vi "UpdateGetTerm.vi"(1 "State In":T1 {"BlockNodeState"."Draw Style" items=["FunctionBlock", "ExpressVI", "Variable", "Elemental I/O", "32x32 Icon", "FunctionBlockCompact"]; "BlockNodeState"."Terminal Data"."Terminal Flags" format="%.0b"}) -> (0 "State Out":T1 {"BlockNodeState"."Draw Style" items=["FunctionBlock", "ExpressVI", "Variable", "Elemental I/O", "32x32 Icon", "FunctionBlockCompact"]; "BlockNodeState"."Terminal Data"."Terminal Flags" format="%.0b"})   [LabVIEW 2017, in "Get DDT Properties.lvlib"]
uses:
  <vilib>/express/express signal manip/GetorSetDDTAttributes/Get DDT Attributes/Get DDT Properties.lvlib
  <vilib>/express/express signal manip/GetorSetDDTAttributes/Get DDT Attributes/State.ctl
  <vilib>/BlockNodeSupport/BlockNodeState.ctl
  <vilib>/BlockNodeSupport/TerminalData.ctl
  <vilib>/picture/picture.llb/imagedata.ctl
  <vilib>/express/express signal manip/GetorSetDDTAttributes/Shared VIs/Attributes data.ctl
  <vilib>/express/express signal manip/GetorSetDDTAttributes/Shared VIs/Input.ctl
  <vilib>/express/express signal manip/GetorSetDDTAttributes/Shared VIs/Attributes name.ctl
  <vilib>/express/express signal manip/GetorSetDDTAttributes/Shared VIs/XDimension.ctl
  <vilib>/express/express signal manip/GetorSetDDTAttributes/Shared VIs/TimeType.ctl
  <vilib>/express/express signal manip/GetorSetDDTAttributes/Shared VIs/GetSetShared.lvlib
  <vilib>/express/express signal manip/GetorSetDDTAttributes/Get DDT Attributes/Get DDT Properties.xnode
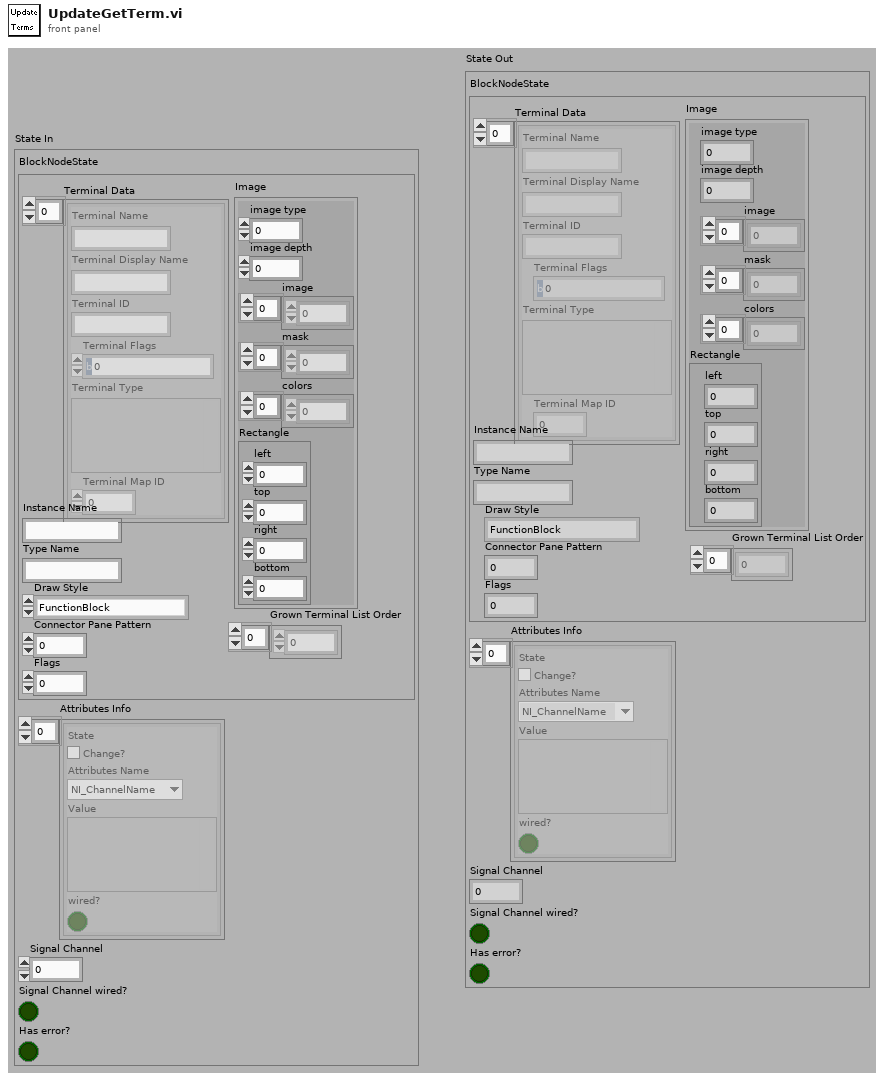
[diagram p1: front panel]
types:
  T1 = typedef "Get DDT Properties.lvlib/Get DDT Properties.xnode/State.ctl" = cluster{"BlockNodeState":T2, "Attributes Info":T5[], "Signal Channel":u32, "Signal Channel wired?":bool, "Has error?":bool}
  T2 = typedef "BlockNodeState.ctl" = cluster{"Terminal Data":T3[], "Instance Name":string, "Type Name":string, "Draw Style":i32, "Connector Pane Pattern":i32, "Flags":i32, "Grown Terminal List Order":i32[], "Image":T4}
  T3 = typedef "TerminalData.ctl" = cluster{"Terminal Name":string, "Terminal Display Name":string, "Terminal ID":string, "Terminal Flags":i32, "Terminal Type":variant, "Terminal Map ID":i32}
  T4 = typedef "imagedata.ctl" = cluster{"image type":i32, "image depth":i32, "image":u8[], "mask":u8[], "colors":u32[], "Rectangle":cluster{"left":i16, "top":i16, "right":i16, "bottom":i16}}
  T5 = typedef "GetSetShared.lvlib/Attributes data.ctl" = cluster{"State":T6, "Attributes Name":T7, "Value":variant, "wired?":bool}
  T6 = typedef "GetSetShared.lvlib/Input.ctl" = bool
  T7 = typedef "GetSetShared.lvlib/Attributes name.ctl" = enum16{"NI_ChannelName", "NI_ExpIsRelativeTime", "NI_ExpTimeStamp", "NI_ExpStartTimeStamp", "NI_ExpXDimension", "NI_UnitDescription"}
  T8 = cluster{"Terminal Name":string, "Terminal Display Name":string, "Terminal ID":string, "Terminal Flags":i32, "Terminal Type":variant, "Terminal Map ID":i32}
  T9 = typedef "GetSetShared.lvlib/XDimension.ctl" = enum16{"No Unit [-]", "Time [sec]", "Frequency [Hz]"}
  T10 = typedef "GetSetShared.lvlib/TimeType.ctl" = enum16{"Absolute", "Relative"}
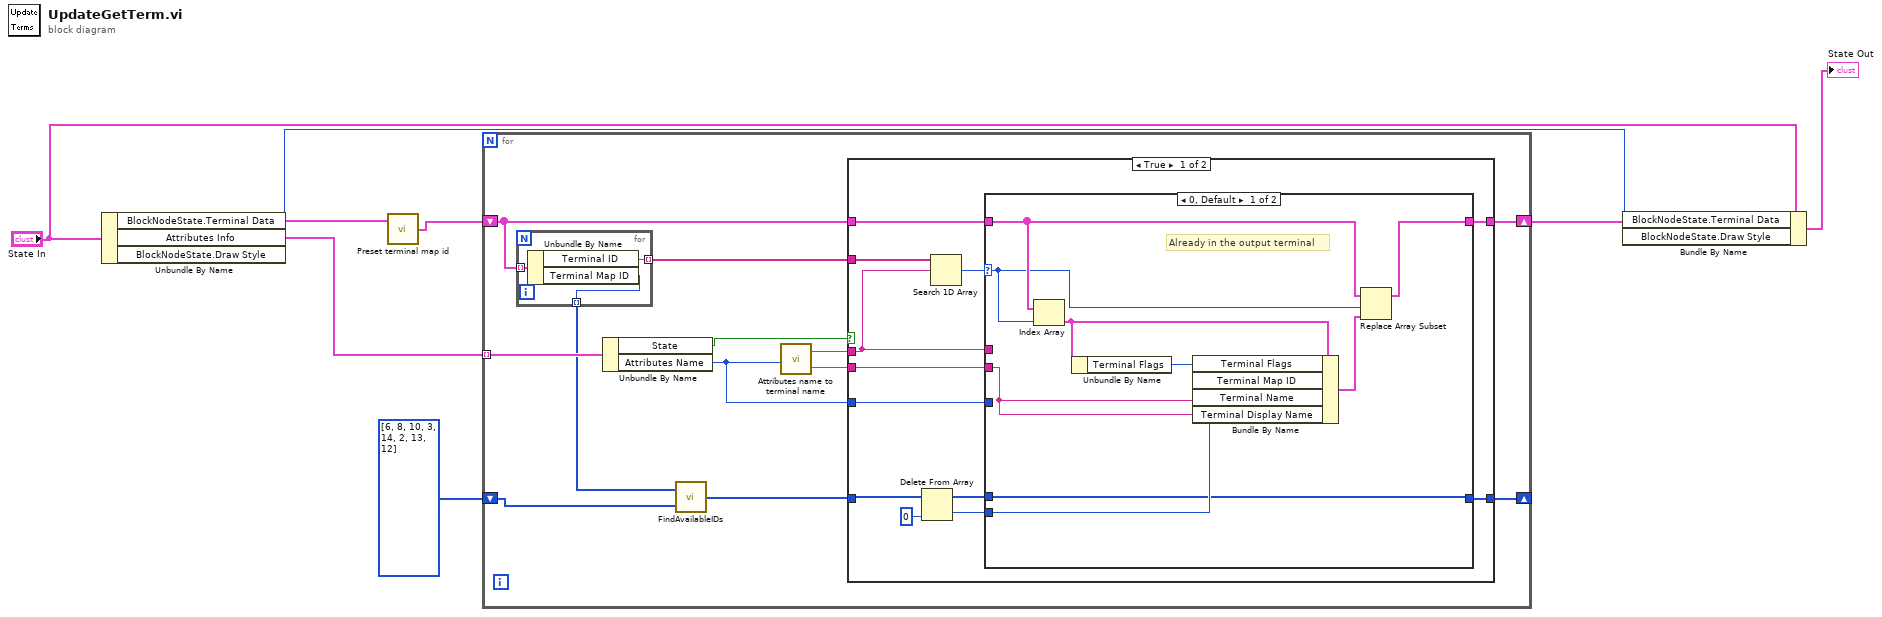
[diagram p0: block diagram]
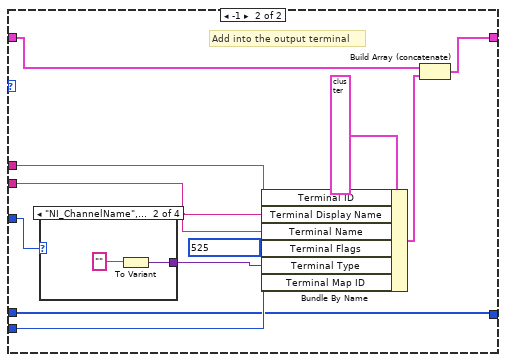
[diagram p2: hidden frame]
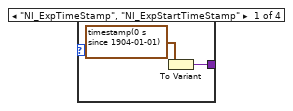
[diagram p3: hidden frame]
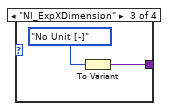
[diagram p4: hidden frame]
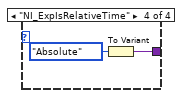
[diagram p5: hidden frame]
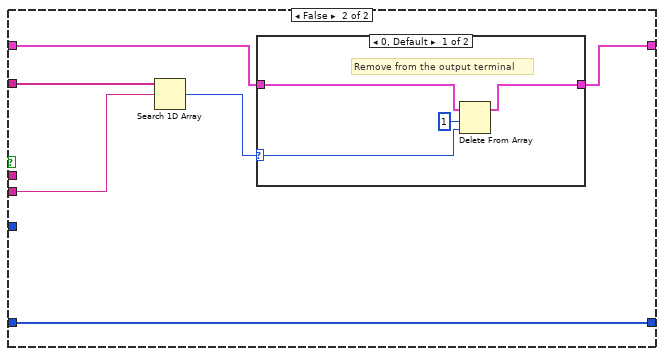
[diagram p6: hidden frame]
diagram:
  n1 = Unbundle By Name("State In") -> ("BlockNodeState.Terminal Data"=w6:T3[], "Attributes Info"=w8:T5[], "BlockNodeState.Draw Style"=w7:i32)
  n2 = call <vilib>:"Preset terminal map id.vi"("Terminal Data in"=w6) -> ("Terminal Data out"=w2:T3[])  [unwired: 1 out]
  n3 = for {
    tunnel: w8 -> [w20] mode=indexing
    shift-right: [w19] -> w3
    shift-left: w2 -> [w17]
    shift-right: [w15] -> _
    shift-left: i32[] [6, 8, 10, 3, 14, 2, 13, 12] ("available map id") -> [w12]
    n4 = for {
      tunnel: w17 -> [w23] mode=indexing
      tunnel: [w22] -> w14 mode=indexing
      tunnel: [w21] -> w11 mode=indexing
      n5 = Unbundle By Name(w23) -> ("Terminal ID"=w22:string, "Terminal Map ID"=w21:i32)
    }
    n6 = Unbundle By Name(w20) -> ("State"=w18:T6, "Attributes Name"=w13:T7)
    n7 = call <vilib>:"FindAvailableIDs.vi"("All ids"=w12, "Unavailable ids"=w11) -> ("available map id"=w10:i32[])
    n8 = call <vilib>:"Attributes name to terminal name.vi"("Attributes Name"=w13) -> ("terminal Name"=w16:string, "Terminal ID"=w9:string)  [unwired: 1 out]
    n9 = case shown="True" w18 {
      tunnel: w17 -> [w34 w66]
      tunnel: [w33 w65] -> w19
      tunnel: w14 -> [w35 w69]
      tunnel: w16 -> [w30 w68]
      tunnel: w13 -> [w31 _]
      tunnel: w10 -> [w27 w64]
      tunnel: [w29 w64] -> w15
      tunnel: w9 -> [w24 _]
      frame True {
        n10 = Delete From Array(array=w27, index=0) -> (deleted portion=w28:i32, array with subset deleted=w25:i32[])  [unwired: 1 in]
        n11 = Search 1D Array(1D array=w35, element=w24) -> (index of element=w32:i32)  [unwired: 1 out]
        n12 = case shown="0, Default" w32 {
          selector: w32 -> [w42 _]
          tunnel: w34 -> [w43 w52]
          tunnel: [w40 w51] -> w33
          tunnel: w31 -> [_ w49]
          tunnel: w30 -> [w37 w50]
          tunnel: w28 -> [w44 w47]
          tunnel: [w39 w46] -> w29
          tunnel: w25 -> [w39 w46]
          tunnel: w24 -> [_ w45]
          frame 0, Default {
            # "Already in the output terminal"
            n13 = Index Array(array=w43, index=w42) -> (element=w38:T3)
            n14 = Unbundle By Name(w38) -> ("Terminal Flags"=w36:i32)
            n15 = Bundle By Name(cluster=w38, "Terminal Flags"=w36, "Terminal Map ID"=w44, "Terminal Name"=w37, "Terminal Display Name"=w37) -> (w41:T3)
            n16 = Replace Array Subset(array=w43, new element=w41, index=w42) -> (w40:T3[])
          }
          frame -1 {
            # "Add into the output terminal"
            n17 = case shown="\"NI_ChannelName\", Default" w49 {
              tunnel: [w57 w59 w61 w63] -> w48
              frame "NI_ExpTimeStamp", "NI_ExpStartTimeStamp" {
                n18 = To Variant(anything=timestamp(0 s since 1904-01-01)) -> (Variant=w57:variant)
              }
              frame "NI_ChannelName", Default {
                n19 = To Variant(anything="") -> (Variant=w59:variant)
              }
              frame "NI_ExpXDimension" {
                n20 = To Variant(anything=XDimension."No Unit [-]" ("XDimension")) -> (Variant=w61:variant)
              }
              frame "NI_ExpIsRelativeTime" {
                n21 = To Variant(anything=TimeType."Absolute" ("RelativeTime?")) -> (Variant=w63:variant)
              }
            }
            n22 = Bundle By Name(cluster=T8 {"Terminal Name"="", "Terminal Display Name"="", "Terminal ID"="", "Terminal Flags"=0, "Terminal Type"=variant, "Terminal Map ID"=0} ("XNTerminalData"), "Terminal ID"=w45, "Terminal Display Name"=w50, "Terminal Name"=w50, "Terminal Flags"=525, "Terminal Type"=w48, "Terminal Map ID"=w47) -> (w53:T8)
            n23 = Build Array (concatenate)(w52, w53) -> (w51:T3[])
          }
        }
      }
      frame False {
        n24 = Search 1D Array(1D array=w69, element=w68) -> (index of element=w67:i32)  [unwired: 1 out]
        n25 = case shown="0, Default" w67 {
          selector: w67 -> [w72 _]
          tunnel: [w70 w74] -> w65
          tunnel: w66 -> [w73 w74]
          frame 0, Default {
            # "Remove from the output terminal"
            n26 = Delete From Array(array=w73, length=1, index=w72) -> (array with subset deleted=w70:T3[])  [unwired: 1 out]
          }
          frame -1 {
            # "not in the output terminal"
          }
        }
      }
    }
  }
  n27 = Bundle By Name(cluster="State In", "BlockNodeState.Terminal Data"=w3, "BlockNodeState.Draw Style"=w7) -> (→"State Out":T1)
